vi "Reachable Time Acceleration.vi"(1 "Max Acceleration":dbl, 2 "Reachable Angular Velocity":dbl) -> (0 "Reachable Time Acceleration":dbl)   [LabVIEW 2015]
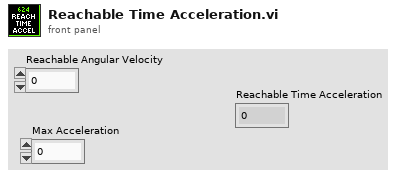
[diagram p1: front panel]
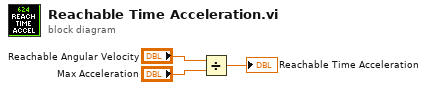
[diagram p0: block diagram]
diagram:
  n1 = Divide(x="Reachable Angular Velocity", y="Max Acceleration") -> (x/y=→"Reachable Time Acceleration":dbl)
